vi "Status.vi"(8 "error in (no error)":errorcluster, 11 "EPOS4 Settings In":T3={"VISA resource name"="", "axis"={"keyHandle"=0, "nodeId"=1}, "Simulated?"=FALSE}) -> (0 "error out":errorcluster, 1 "Connection Error":bool, 2 "Centrifuge On?":enum16{"Off", "On", "Not Initialized"}(ring), 3 "EPOS4 Settings Out":T3={"VISA resource name"="", "axis"={"keyHandle"=0, "nodeId"=1}, "Simulated?"=FALSE}, 5 "axis data":T1)   [LabVIEW 2018, in "EPOS4.lvlib"]
uses:
  Controls/EPOS Communication Settings.ctl
  EPOS4.lvlib
panel:
  out "axis state":T2(ring)
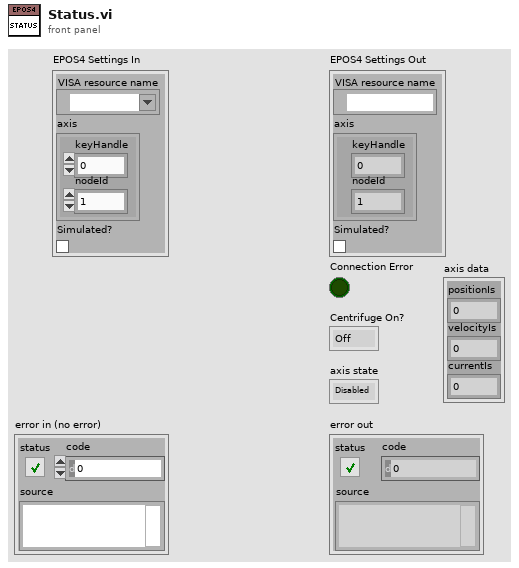
[diagram p1: front panel]
types:
  T1 = cluster{"positionIs":i32, "velocityIs":i32, "currentIs":i16}
  T2 = enum16{"Disabled", "Enabled", "Quickstop", "Fault"}
  T3 = typedef "EPOS4.lvlib/EPOS Communication Settings.ctl" = cluster{"VISA resource name":refnum<visa-resource-name>, "axis":cluster{"keyHandle":u32, "nodeId":u16}, "Simulated?":bool}
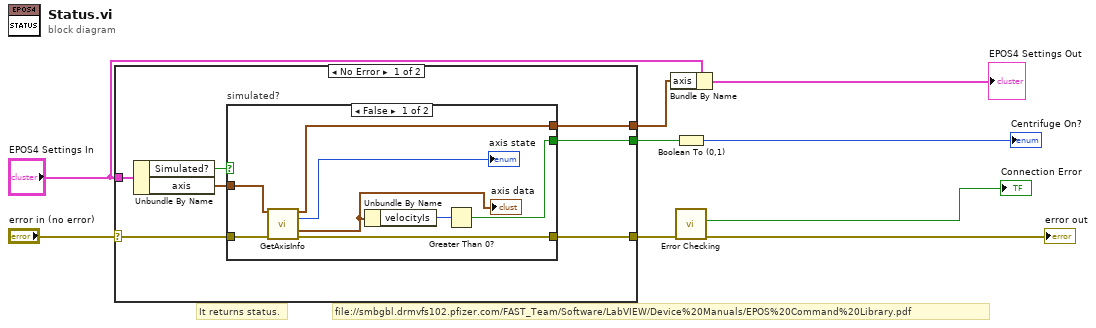
[diagram p0: block diagram]
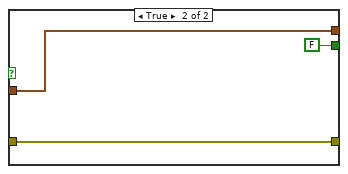
[diagram p2: hidden frame]
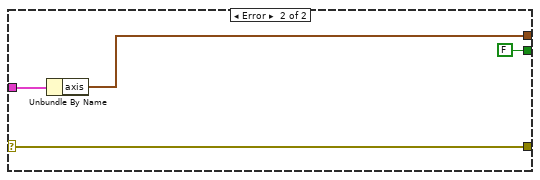
[diagram p3: hidden frame]
diagram:
  # "file://smbgbl.drmvfs102.pfizer.com/FAST_Team/Software/LabVIEW/Device%20Manuals/EPOS%20Command%20Library.pdf"
  # "It returns status."
  n1 = case shown="No Error" "error in (no error)" {
    selector: "error in (no error)" -> [w11 w31]
    tunnel: [w15 w31] -> w8
    tunnel: "EPOS4 Settings In" -> [w14 w29]
    tunnel: [w10 FALSE] -> w5
    tunnel: [w12 w28] -> w1
    frame No Error {
      n2 = Unbundle By Name(w14) -> ("Simulated?"=w16:bool, "axis"=w13:cluster{"keyHandle":u32, "nodeId":u16})
      n3 = case "simulated?" shown="False" w16 {
        tunnel: [w17 w26] -> w15
        tunnel: [w22 w25] -> w12
        tunnel: w13 -> [w24 w25]
        tunnel: w11 -> [w23 w26]
        tunnel: [w19 FALSE] -> w10
        frame False {
          n4 = call "GetAxisInfo.vi"("axis in"=w24, "error in (no error)"=w23) -> ("axis out"=w22:cluster{"keyHandle":u32, "nodeId":u16}, "axis state"=→"axis state":T2, "axis data"=w20:T1, "error out"=w17:errorcluster)  [unwired: 9 in, 1 out]
          "axis data" <- w20
          n5 = Unbundle By Name(w20) -> ("velocityIs"=w18:i32)
          n6 = Greater Than 0?(x=w18) -> (x > 0?=w19:bool)
        }
        frame True {
        }
      }
    }
    frame Error {
      n7 = Unbundle By Name(w29) -> ("axis"=w28:cluster{"keyHandle":u32, "nodeId":u16})
    }
  }
  n8 = Bundle By Name(cluster="EPOS4 Settings In", "axis"=w1) -> (→"EPOS4 Settings Out":T3)
  n9 = Boolean To (0,1)(Boolean=w5) -> (0, 1=→"Centrifuge On?":i16)
  n10 = call "Error Checking.vi"("error in (no error)"=w8) -> ("error out"=→"error out":errorcluster, "Connection Error"=→"Connection Error":bool)  [unwired: 8 in, 1 out]
